vi "GetDataEvent_Service_3.vi"() -> ()   [LabVIEW 2017]
doc: "This is an example of how to read Data Sets from the InsightCM database. Using a similiar method you can read any waveform that has been stored and perform additional analysis on it or save it to a file format."
uses:
  <vilib>/addons/InsightCM/MessageBus/Base/controls/AssetNodeView.ctl
  <vilib>/addons/InsightCM/MessageBus/Base/controls/AssetState.ctl
  <vilib>/addons/InsightCM/MessageBus/Base/controls/Metric.ctl
  <vilib>/addons/InsightCM/MessageBus/Base/controls/KeyValuePair.ctl
  <vilib>/addons/InsightCM/MessageBus/Base/controls/AssetNodeReference.ctl
  <vilib>/addons/InsightCM/MessageBus/Base/controls/DataEvent.ctl
  <vilib>/addons/InsightCM/MessageBus/Base/controls/DataSetByteData.ctl
  <vilib>/addons/InsightCM/MessageBus/Base/controls/TrendPoint.ctl
  typedefs/Asset Info.ctl
  typedefs/Sensor Info.ctl
  typedefs/Metric Info.ctl
  typedefs/Q_Message.ctl
  typedefs/Input IDs.ctl
  <vilib>/addons/InsightCM/MessageBus/MessageService/IcmMessageService.lvclass
panel:
  out "element":T1
  out "Output 2":T2(array[cluster])
  out "DataEvents 2":T3[](array[typedef])=[{"Id"="{6C8D9120-E97A-11E9-9C35-00802F195E7B}", "AssetNodeId"="5cf73cf3a0991c03a125caeb", "Timestamp"=1570418361, "Props"=[{"Key"="DeviceName", "Value"="John-9068"}, {"Key"="DataGroup", "Value"="Equipment"}, {"Key"="OpState", "Value"="Default"}, {"Key"="Reason", "Value"="User Event"}, {"Key"="HighRate", "Value"="true"}, {"Key"="HasDataSets", "Value"="true"}]}, {"Id"="{7F637499-E981-11E9-A30F-00802F195E7B}", "AssetNodeId"="5cf73cf3a0991c03a125caeb", "Timestamp"=1570421399, "Props"=[{"Key"="DeviceName", "Value"="John-9068"}, {"Key"="DataGroup", "Value"="Equipment"}, {"Key"="OpState", "Value"="Default"}, {"Key"="Reason", "Value"="Periodic Event"}, {"Key"="HighRate", "Value"="true"}, {"Key"="HasDataSets", "Value"="true"}]}, {"Id"="{E4F320D8-E982-11E9-A025-00802F195E7B}", "AssetNodeId"="5cf73cf3a0991c03a125caeb", "Timestamp"=1570421999, "Props"=[{"Key"="DeviceName", "Value"="John-9068"}, {"Key"="DataGroup", "Value"="Equipment"}, {"Key"="OpState", "Value"="Default"}, {"Key"="Reason", "Value"="Periodic Event"}, {"Key"="HighRate", "Value"="true"}, {"Key"="HasDataSets", "Value"="true"}]}, {"Id"="{97B5DB2B-E983-11E9-8698-00802F195E7B}", "AssetNodeId"="5cf73cf3a0991c03a125caeb", "Timestamp"=1570422299, "Props"=[{"Key"="DeviceName", "Value"="John-9068"}, {"Key"="DataGroup", "Value"="Equipment"}, {"Key"="OpState", "Value"="Default"}, {"Key"="Reason", "Value"="Periodic Event"}, {"Key"="HighRate", "Value"="true"}, {"Key"="HasDataSets", "Value"="true"}]}, {"Id"="{FD7A4AB0-E984-11E9-A552-00802F195E7B}", "AssetNodeId"="5cf73cf3a0991c03a125caeb", "Timestamp"=1570422899, "Props"=[{"Key"="DeviceName", "Value"="John-9068"}, {"Key"="DataGroup", "Value"="Equipment"}, {"Key"="OpState", "Value"="Default"}, {"Key"="Reason", "Value"="Periodic Event"}, {"Key"="HighRate", "Value"="true"}, {"Key"="HasDataSets", "Value"="true"}]}, {"Id"="{B025F119-E985-11E9-9683-00802F195E7B}", "AssetNodeId"="5cf73cf3a0991c03a125caeb", "Timestamp"=1570423199, "Props"=[{"Key"="DeviceName", "Value"="John-9068"}, {"Key"="DataGroup", "Value"="Equipment"}, {"Key"="OpState", "Value"="Default"}, {"Key"="Reason", "Value"="Periodic Event"}, {"Key"="HighRate", "Value"="true"}, {"Key"="HasDataSets", "Value"="true"}]}, {"Id"="{62F87800-E986-11E9-9683-00802F195E7B}", "AssetNodeId"="5cf73cf3a0991c03a125caeb", "Timestamp"=1570423499, "Props"=[{"Key"="DeviceName", "Value"="John-9068"}, {"Key"="DataGroup", "Value"="Equipment"}, {"Key"="OpState", "Value"="Default"}, {"Key"="Reason", "Value"="Periodic Event"}, {"Key"="HighRate", "Value"="true"}, {"Key"="HasDataSets", "Value"="true"}]}]
  out "LastTrendPoint":cluster{string, "Value":dbl}
  in  "String":string="This is an EXE to host a web service for InsightCM.\n\nhttp://127.0.0.1:8002/Query/GetLastEvent?Asset=<AssetName>\nOutput: Last event for the asset within X days, all channels (JSON)\n\nhttp://127.0.0.1:8002/Query/GetAssetList\nOutput: Asset ID, Sensor ID, and Metric ID (JSON)\n\nhttp://127.0.0.1:8002/Query/GetLastTrend?MetricID=<Metric ID of feature>\nOutput: Time and value of last trend point (JSON)\n\nhttp://127.0.0.1:8002/Query/GetEventList?FID_2={value}&FID_1={value}&SensorID={value}&AssetID={value}\nOutput: From asset and sensor, give list of recent event waveform and feature data (JSON)\n\nhttp://127.0.0.1:8002/Query/GetEvent?FID_2={value}&FID_1={value}&SensorID={value}&AssetID={value}\nOutput: From asset and sensor, give most recent event waveform and feature data (JSON)"
  out "Trend":T5(graph)
  out "SIGMU Output":T6[](array[typedef])
  in  "Seconds from now":i64=3600
  out "error out":errorcluster
  out "Ready?":bool
  out "Parameter (debug)":string
  out "Command (debug)":string
  out "Output":T9(array[cluster])
  out "TrendPoints":T10[](array[typedef])
  out "DataSets":T11[](array[typedef])
  out "date/time":string
  out "Numeric":i32
  out "DataEvents":T3[](array[typedef])
  out "AssetNodeView":T12
  out "AssetNodes":T12[](array[typedef])
  # "1 hr = 3600, 1 day = 86400"
  # "This example shows how to query InsightCM data.\n\n1) Click Refresh to load assets.\n2) Select an asset.\n3) Select a data event and a sensor.\n\nNote: If the sensor does not have waveform data, the waveform graph will be empty."
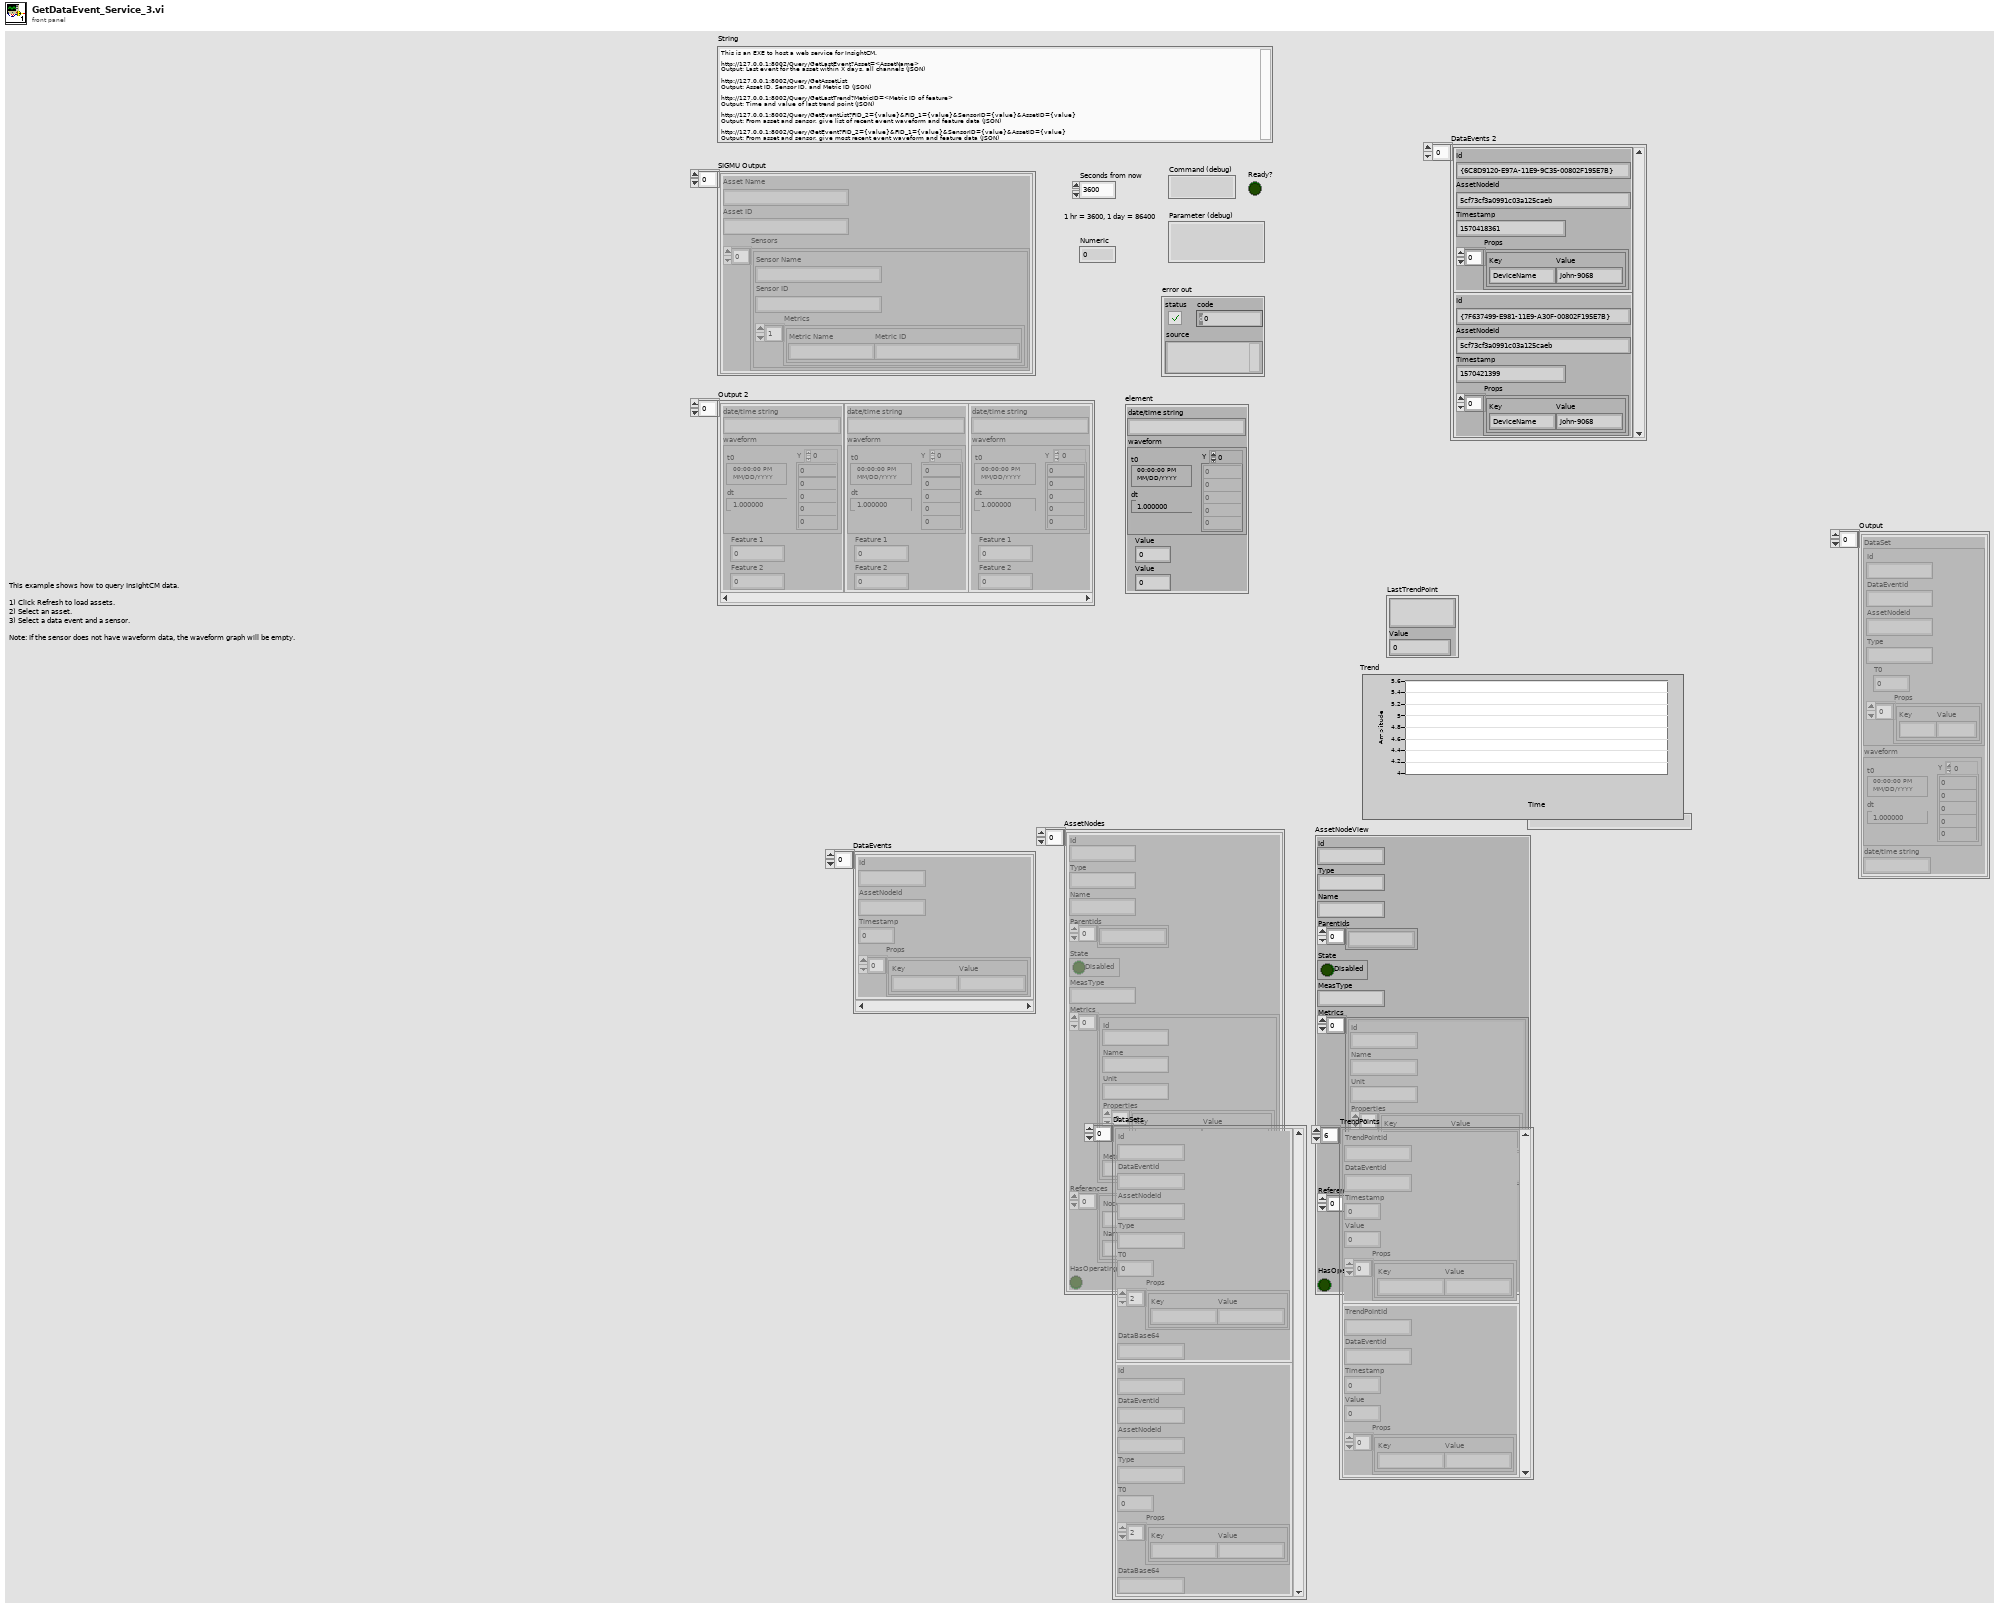
[diagram p1: front panel]
types:
  T1 = cluster{"date/time string":string, "waveform":waveform(sgl), "Value":dbl, "Value":dbl}
  T2 = cluster{"date/time string":string, "waveform":waveform(sgl), "Feature 1":dbl, "Feature 2":dbl}[]
  T3 = typedef "DataEvent.ctl" = cluster{"Id":string, "AssetNodeId":string, "Timestamp":i64, "Props":T4[]}
  T4 = typedef "KeyValuePair.ctl" = cluster{"Key":string, "Value":string}
  T5 = cluster{"Time Stamp out":timestamp, "Value":dbl}[]
  T6 = typedef "Asset Info.ctl" = cluster{"Asset Name":string, "Asset ID":string, "Sensors":T7[]}
  T7 = typedef "Sensor Info.ctl" = cluster{"Sensor Name":string, "Sensor ID":string, "Metrics":T8[]}
  T8 = typedef "Metric Info.ctl" = cluster{"Metric Name ":string, "Metric ID":string}
  T9 = cluster{"DataSet":cluster{"Id":string, "DataEventId":string, "AssetNodeId":string, "Type":string, "T0":i64, "Props":T4[]}, "waveform":waveform(sgl), "date/time string":string}[]
  T10 = typedef "TrendPoint.ctl" = cluster{"TrendPointId":string, "DataEventId":string, "Timestamp":i64, "Value":dbl, "Props":T4[]}
  T11 = typedef "DataSetByteData.ctl" = cluster{"Id":string, "DataEventId":string, "AssetNodeId":string, "Type":string, "T0":i64, "Props":T4[], "DataBase64":string}
  T12 = typedef "AssetNodeView.ctl" = cluster{"Id":string, "Type":string, "Name":string, "ParentIds":string[], "State":T13, "MeasType":string, "Metrics":T14[], "References":T15[], "HasOperatingStates":bool}
  T13 = typedef "AssetState.ctl" = cluster{"Disabled":bool}
  T14 = typedef "Metric.ctl" = cluster{"Id":string, "Name":string, "Unit":string, "Properties":T4[], "MetricDefinitionInstanceId":string}
  T15 = typedef "AssetNodeReference.ctl" = cluster{"NodeId":string, "Name":string}
  T16 = typedef "Q_Message.ctl" = cluster{"Command":string, "Parameters":variant}
  T17 = cluster{"Id":string, "DataEventId":string, "AssetNodeId":string, "Type":string, "T0":i64, "Props":T4[]}
  T18 = cluster{"DataSet":cluster{"Id":string, "DataEventId":string, "AssetNodeId":string, "Type":string, "T0":i64, "Props":T4[]}, "waveform":waveform(sgl), "date/time string":string}
  T19 = typedef "Input IDs.ctl" = cluster{"Asset ID":string, "Sensor ID":string, "Feature id 1":string, "Feature id 2":string}
  T20 = cluster{"date/time string":string, "waveform":waveform(sgl), "Value":dbl, "Value":dbl}[]
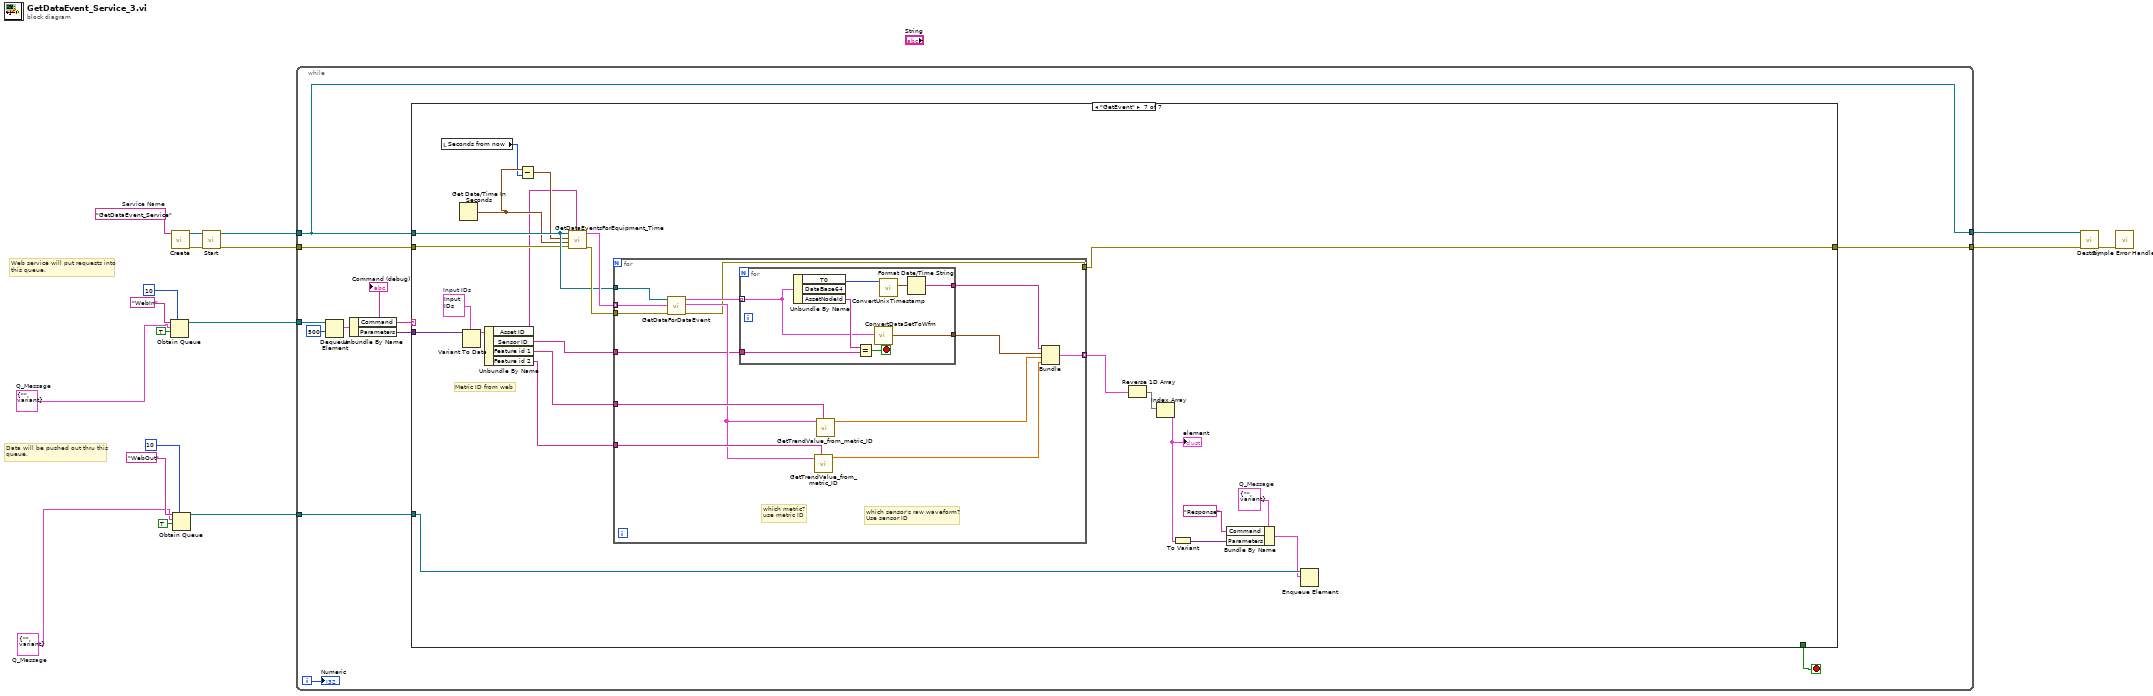
[diagram p0: block diagram]
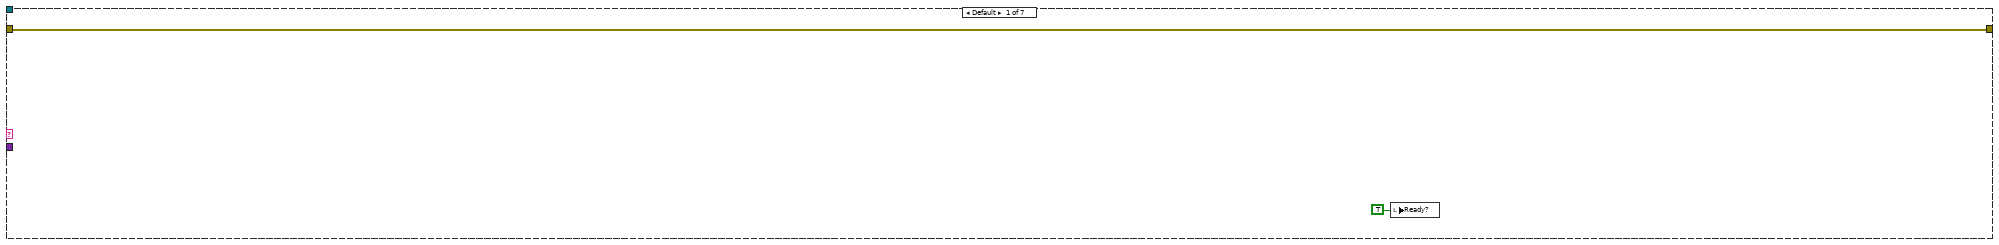
[diagram p2: hidden frame]
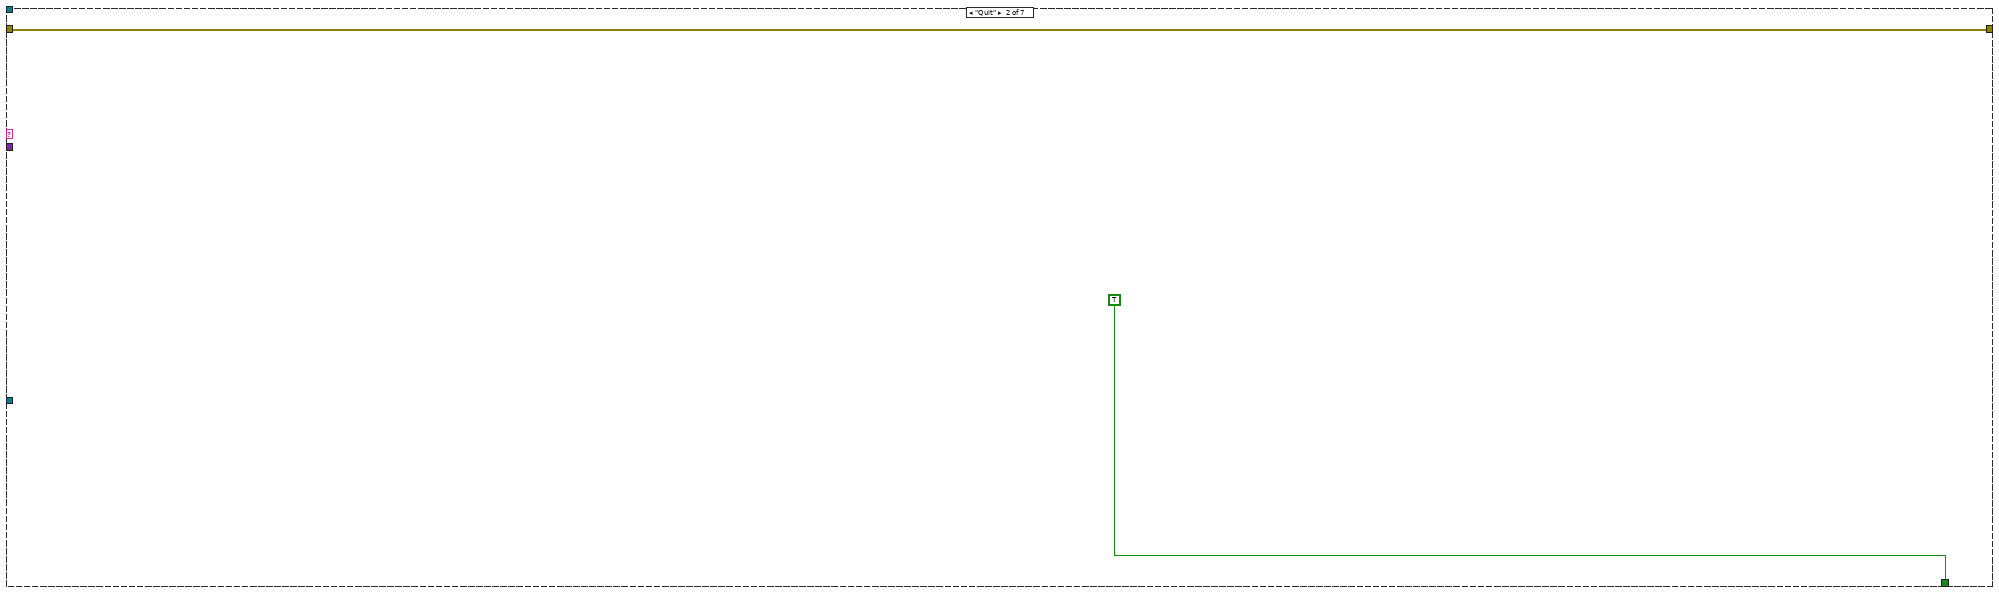
[diagram p3: hidden frame]
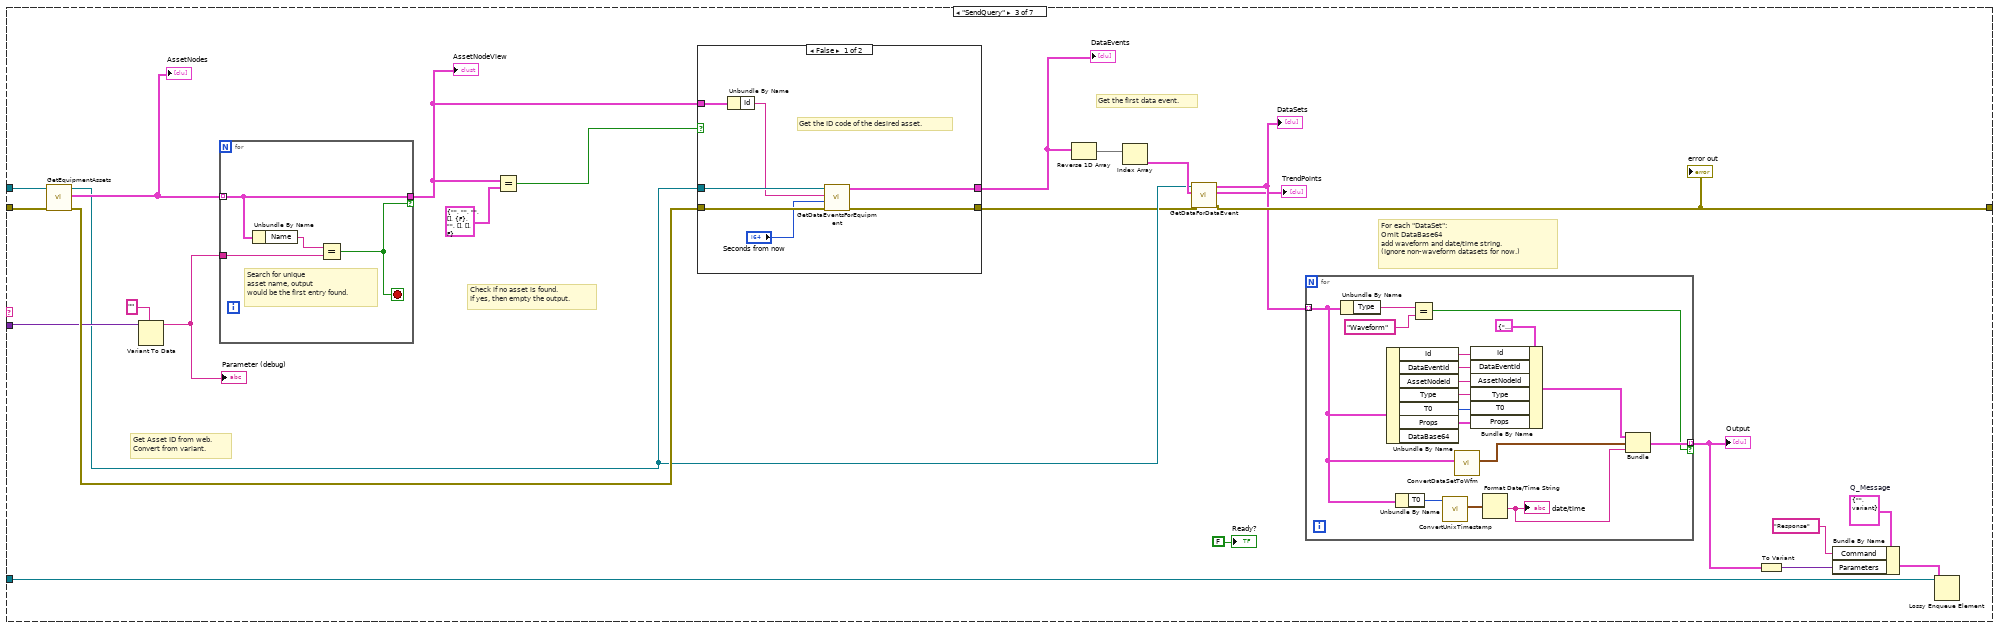
[diagram p4: hidden frame]
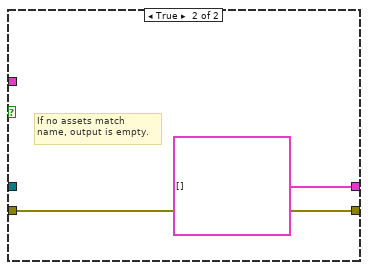
[diagram p5: hidden frame]
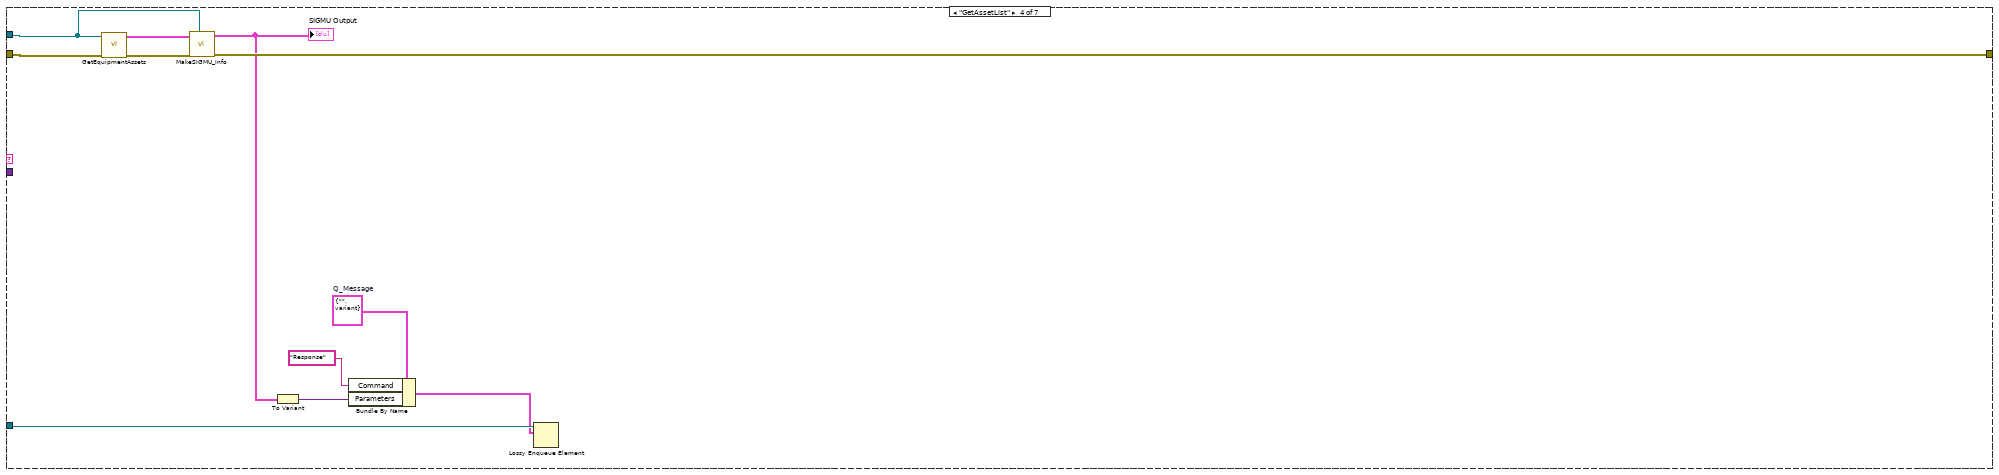
[diagram p6: hidden frame]
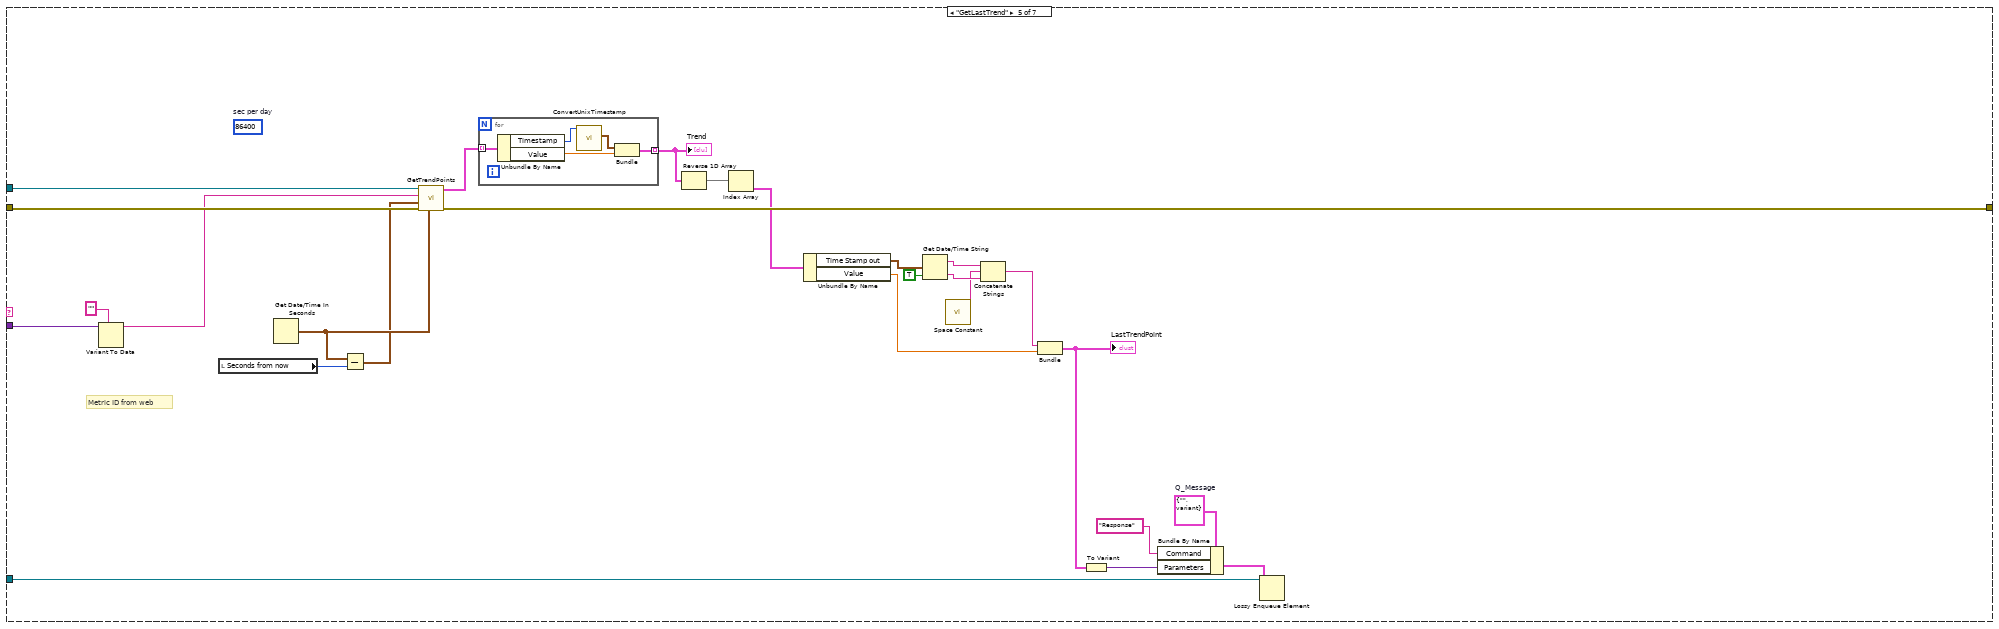
[diagram p7: hidden frame]
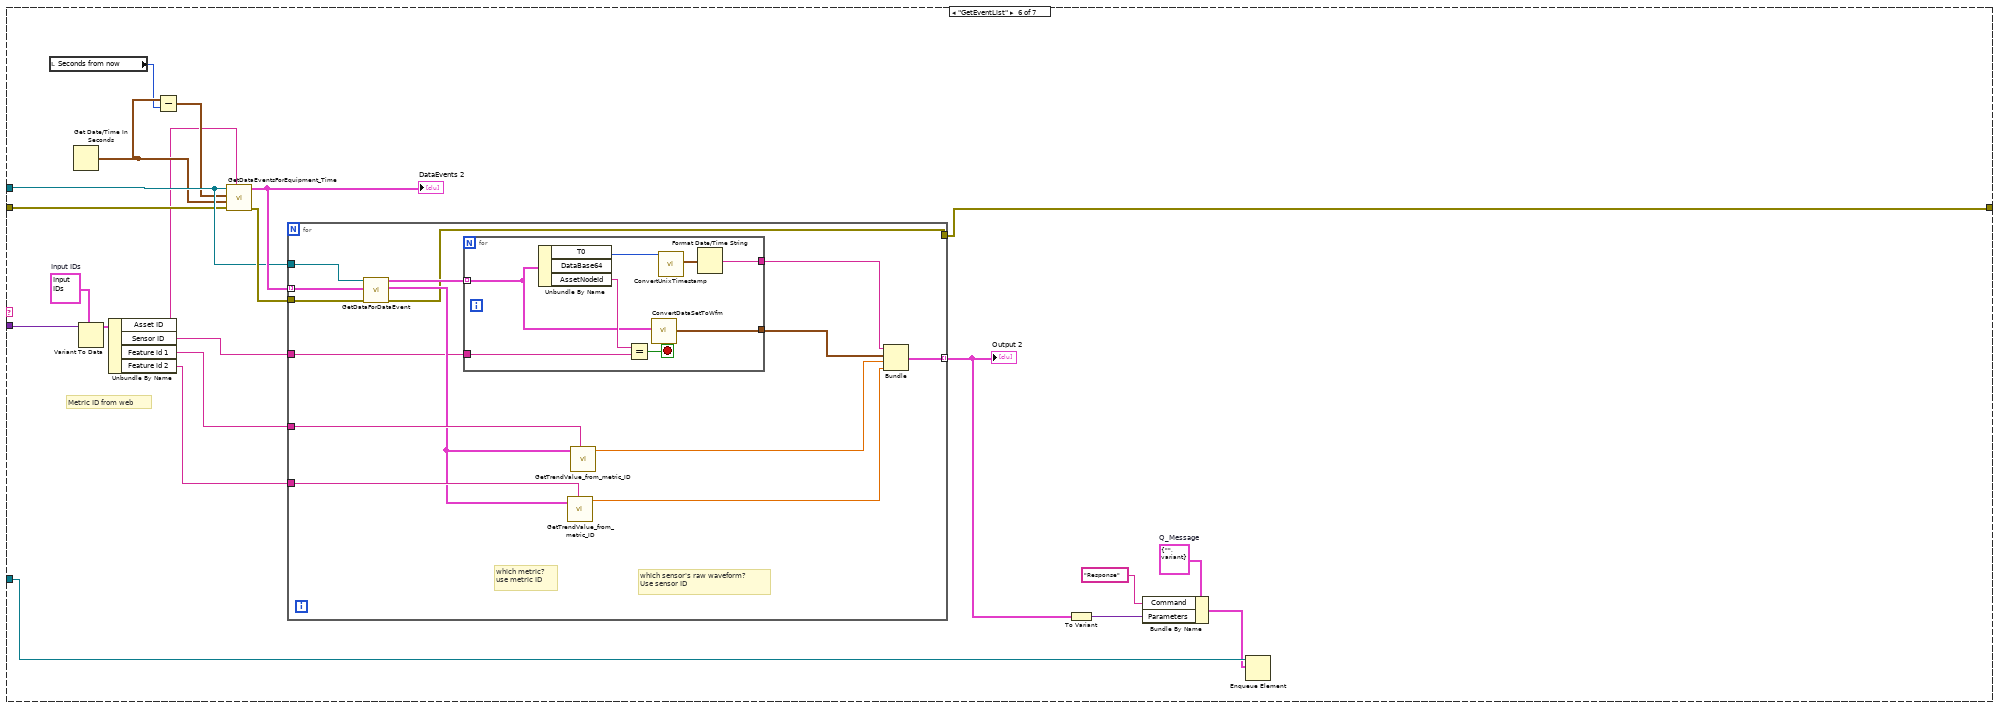
[diagram p8: hidden frame]
diagram:
  w1 = T16 {"Command"="", "Parameters"=variant}  # Q_Message
  w2 = T16 {"Command"="", "Parameters"=variant}  # Q_Message
  w18 = "GetDataEvent_Service"  # Service Name
  # "Data will be pushed out thru this\nqueue."
  # "Web service will put requests into\nthis queue."
  n1 = Obtain Queue(max queue size (-1, unlimited)=10, name (unnamed)="WebIn", element data type=w2, create if not found? (T)=TRUE) -> (queue out=w8:refnum<queue>)  [unwired: 1 in, 2 out]
  n2 = call <vilib>:"Create.vi"("service name"=w18) -> ("error out"=w13:errorcluster, "service out"=w14:refnum<class "IcmMessageService.lvclass">)  [unwired: 9 in]
  n3 = Obtain Queue(max queue size (-1, unlimited)=10, name (unnamed)="WebOut", element data type=w1, create if not found? (T)=TRUE) -> (queue out=w7:refnum<queue>)  [unwired: 1 in, 2 out]
  n4 = call <vilib>:"Start.vi"("error in (no error)"=w13, "service in"=w14) -> ("error out"=w11:errorcluster, "service out"=w12:refnum<class "IcmMessageService.lvclass">)  [unwired: 8 in]
  n5 = while {
    tunnel: w12 -> [w28]
    tunnel: w11 -> [w29]
    tunnel: [w28] -> w15
    tunnel: [w27] -> w16
    tunnel: w8 -> [w26]
    tunnel: w7 -> [w24]
    i -> [w19]
    stop <- w23 stop-if-true
    n6 = Dequeue Element(queue=w26, timeout in ms (-1)=500) -> (element=w22:T16)  [unwired: 1 in, 3 out]
    n7 = Unbundle By Name(w22) -> ("Command"=w21:string, "Parameters"=w20:variant)
    "Command (debug)" <- w21
    n8 = case shown="\"GetEvent\"" w21 {
      tunnel: w29 -> [w31 w33 w57 w98 w122 w147 w192]
      tunnel: w28 -> [_ _ w45 w96 w123 w148 w193]
      tunnel: [w31 w33 w43 w94 w115 w130 w176] -> w27
      tunnel: w24 -> [_ _ w36 w90 w108 w136 w181]
      tunnel: [_ TRUE _ _ _ _ _] -> w23
      tunnel: w20 -> [_ _ w51 _ w120 w146 w191]
      frame Default {
        n9 = local write "Ready?"(TRUE ("Ready?")) -> ()
      }
      frame "Quit" {
      }
      frame "SendQuery" {
        w34 = T16 {"Command"="", "Parameters"=variant}  # Q_Message
        # "For each \"DataSet\":\nOmit DataBase64\nadd waveform and date/time string.\n(Ignore non-waveform datasets for now.)"
        # "Get Asset ID from web.\nConvert from variant."
        # "Get the first data event."
        # "Check if no asset is found.\nIf yes, then empty the output."
        n10 = call "GetEquipmentAssets.vi"("error in (no error)"=w57, "service"=w45) -> ("error out"=w53:errorcluster, "AssetNodes"=w56:T12[])  [unwired: 8 in]
        "AssetNodes" <- w56
        n11 = Variant To Data(type="", Variant=w51) -> (data=w49:string)  [unwired: 1 in, 1 out]
        "Parameter (debug)" <- w49
        n12 = for {
          tunnel: w56 -> [w85] mode=indexing
          tunnel: w49 -> [w86]
          tunnel: [w85] -> w54 if=w84
          stop <- w84 stop-if-true
          # "Search for unique \nasset name, output\nwould be the first entry found."
          n13 = Unbundle By Name(w85) -> ("Name"=w87:string)
          n14 = Equal?(x=w87, y=w86) -> (x = y?=w84:bool)
        }
        "AssetNodeView" <- w54
        n15 = Equal?(x=w54, y=T12 {"Id"="", "Type"="", "Name"="", "ParentIds"=[], "State"={"Disabled"=FALSE}, "MeasType"="", "Metrics"=[], "References"=[], "HasOperatingStates"=FALSE} ("AssetNodeView 2")) -> (x = y?=w52:bool)
        n16 = case shown="False" w52 {
          tunnel: w54 -> [w79 _]
          tunnel: w45 -> [w81 _]
          tunnel: w53 -> [w80 w82]
          tunnel: [w78 T3[] [] ("DataEvents")] -> w48
          tunnel: [w77 w82] -> w44
          frame False {
            # "Get the ID code of the desired asset."
            n17 = Unbundle By Name(w79) -> ("Id"=w76:string)
            n18 = call "GetDataEventsForEquipment.vi"("error in (no error)"=w80, "sec per day"="Seconds from now", "equipment id"=w76, "service"=w81) -> ("error out"=w77:errorcluster, "DataEvents"=w78:T3[])  [unwired: 6 in]
          }
          frame True {
            # "If no assets match\nname, output is empty."
          }
        }
        "DataEvents" <- w48
        n19 = Reverse 1D Array(array=w48) -> (reversed array=w47:T3[])
        n20 = Index Array(array=w47) -> (element=w46:T3)  [unwired: 1 in]
        n21 = call "GetDataForDataEvent.vi"("error in (no error)"=w44, "DataEvent"=w46, "service"=w45) -> ("error out"=w43:errorcluster, "TrendPoints"=→"TrendPoints":T10[], "DataSets"=w42:T11[])  [unwired: 6 in]
        "DataSets" <- w42
        "error out" <- w43
        n22 = for {
          tunnel: w42 -> [w66] mode=indexing
          tunnel: [w68] -> w35 mode=indexing if=w67
          n23 = Unbundle By Name(w66) -> ("Type"=w74:string)
          n24 = Unbundle By Name(w66) -> ("Id"=w64:string, "DataEventId"=w60:string, "AssetNodeId"=w61:string, "Type"=w62:string, "T0"=w63:i64, "Props"=w59:T4[])  [unwired: 1 out]
          n25 = Unbundle By Name(w66) -> ("T0"=w72:i64)
          n26 = Equal?(x=w74, y="Waveform") -> (x = y?=w67:bool)
          n27 = call <vilib>:"ConvertUnixTimestamp.vi"("Timestamp in"=w72) -> ("Time Stamp out"=w71:timestamp)  [unwired: 10 in]
          n28 = call "ConvertDataSetToWfm.vi"("DataSet"=w66) -> ("waveform"=w70:waveform(sgl))  [unwired: 10 in]
          n29 = Bundle By Name(cluster=T17 {"Id"="", "DataEventId"="", "AssetNodeId"="", "Type"="", "T0"=0, "Props"=[]} ("DataSet"), "Id"=w64, "DataEventId"=w60, "AssetNodeId"=w61, "Type"=w62, "T0"=w63, "Props"=w59) -> (w58:T17)
          n30 = Format Date/Time String(seconds (now)=w71) -> (date/time string=w69:string)  [unwired: 2 in]
          "date/time" <- w69
          n31 = Bundle("DataSet"=w58, "waveform"=w70, "date/time string"=w69) -> (w68:T18)  [unwired: 1 in]
        }
        "Output" <- w35
        n32 = To Variant(anything=w35) -> (Variant=w38:variant)
        n33 = Bundle By Name(cluster=w34, "Command"="Response", "Parameters"=w38) -> (w37:T16)
        n34 = Lossy Enqueue Element(queue=w36, element=w37) -> ()  [unwired: 1 in, 4 out]
        "Ready?" <- FALSE ("Ready?")
      }
      frame "GetAssetList" {
        w88 = T16 {"Command"="", "Parameters"=variant}  # Q_Message
        n35 = call "GetEquipmentAssets.vi"("error in (no error)"=w98, "service"=w96) -> ("error out"=w95:errorcluster, "AssetNodes"=w97:T12[])  [unwired: 8 in]
        n36 = call "MakeSIGMU_Info.vi"("ICM Service in"=w96, "error in (no error)"=w95, "AssetNodes In"=w97) -> ("error out"=w94:errorcluster, "SIGMU Output"=w93:T6[])  [unwired: 7 in]
        "SIGMU Output" <- w93
        n37 = To Variant(anything=w93) -> (Variant=w91:variant)
        n38 = Bundle By Name(cluster=w88, "Command"="Response", "Parameters"=w91) -> (w89:T16)
        n39 = Lossy Enqueue Element(queue=w90, element=w89) -> ()  [unwired: 1 in, 4 out]
      }
      frame "GetLastTrend" {
        w109 = T16 {"Command"="", "Parameters"=variant}  # Q_Message
        (unwired) 86400  # sec per day
        # "Metric ID from web"
        n40 = Variant To Data(type="", Variant=w120) -> (data=w119:string)  [unwired: 1 in, 1 out]
        n41 = local read "Seconds from now"() -> (w117:i64)
        n42 = Get Date/Time In Seconds() -> (seconds since 1Jan1904=w118:timestamp)
        n43 = Subtract(x=w118, y=w117) -> (x-y=w116:timestamp)
        n44 = call "GetTrendPoints.vi"("End Time"=w118, "error in (no error)"=w122, "Start Time"=w116, "trend id"=w119, "service"=w123) -> ("error out"=w115:errorcluster, "TrendPoints"=w124:T10[])  [unwired: 5 in]
        n45 = for {
          tunnel: w124 -> [w129] mode=indexing
          tunnel: [w128] -> w113 mode=indexing
          n46 = Unbundle By Name(w129) -> ("Timestamp"=w126:i64, "Value"=w127:dbl)
          n47 = call <vilib>:"ConvertUnixTimestamp.vi"("Timestamp in"=w126) -> ("Time Stamp out"=w125:timestamp)  [unwired: 10 in]
          n48 = Bundle("Time Stamp out"=w125, "Value"=w127) -> (w128:cluster{"Time Stamp out":timestamp, "Value":dbl})  [unwired: 1 in]
        }
        "Trend" <- w113
        n49 = Reverse 1D Array(array=w113) -> (reversed array=w114:T5)
        n50 = Index Array(array=w114) -> (element=w100:cluster{"Time Stamp out":timestamp, "Value":dbl})  [unwired: 1 in]
        n51 = Unbundle By Name(w100) -> ("Time Stamp out"=w107:timestamp, "Value"=w101:dbl)
        n52 = Get Date/Time String(seconds (now)=w107, want seconds? (F)=TRUE) -> (date string=w105:string, time string=w104:string)  [unwired: 1 in]
        n53 = call <vilib>:"Space Constant.vi"() -> ("String"=w103:string)
        n54 = Concatenate Strings(w105, w103, w104) -> (w102:string)
        n55 = Bundle(w102, "Value"=w101) -> (w99:cluster{string, "Value":dbl})  [unwired: 1 in]
        "LastTrendPoint" <- w99
        n56 = To Variant(anything=w99) -> (Variant=w111:variant)
        n57 = Bundle By Name(cluster=w109, "Command"="Response", "Parameters"=w111) -> (w110:T16)
        n58 = Lossy Enqueue Element(queue=w108, element=w110) -> ()  [unwired: 1 in, 4 out]
      }
      frame "GetEventList" {
        w133 = T16 {"Command"="", "Parameters"=variant}  # Q_Message
        w142 = T19 {"Asset ID"="5cf73cf3a0991c03a125caeb", "Sensor ID"="5cf73d1ba0991c03a125caee", "Feature id 1"="5cf73d1ba0991c03a125caef", "Feature id 2"="5cf73d1ba0991c03a125caf0"}  # Input IDs
        # "Metric ID from web"
        n59 = local read "Seconds from now"() -> (w144:i64)
        n60 = Get Date/Time In Seconds() -> (seconds since 1Jan1904=w145:timestamp)
        n61 = Variant To Data(type=w142, Variant=w146) -> (data=w141:T19)  [unwired: 1 in, 1 out]
        n62 = Unbundle By Name(w141) -> ("Asset ID"=w140:string, "Sensor ID"=w137:string, "Feature id 1"=w138:string, "Feature id 2"=w139:string)
        n63 = Subtract(x=w145, y=w144) -> (x-y=w143:timestamp)
        n64 = call "GetDataEventsForEquipment_Time.vi"("equipment id"=w140, "error in (no error)"=w147, "End Time"=w145, "Start Time"=w143, "service"=w148) -> ("error out"=w150:errorcluster, "DataEvents"=w149:T3[])  [unwired: 5 in]
        "DataEvents 2" <- w149
        n65 = for {
          tunnel: w148 -> [w164]
          tunnel: w150 -> [w163]
          tunnel: w149 -> [w162] mode=indexing
          tunnel: [w157] -> w132 mode=indexing
          tunnel: w138 -> [w156]
          tunnel: w139 -> [w155]
          tunnel: w137 -> [w152]
          tunnel: [w151] -> w130
          # "which metric?\nuse metric ID"
          # "which sensor's raw waveform?\nUse sensor ID"
          n66 = call "GetDataForDataEvent.vi"("error in (no error)"=w163, "DataEvent"=w162, "service"=w164) -> ("error out"=w151:errorcluster, "TrendPoints"=w154:T10[], "DataSets"=w161:T11[])  [unwired: 6 in]
          n67 = for {
            tunnel: w161 -> [w167] mode=indexing
            tunnel: w152 -> [w171]
            tunnel: [w166] -> w160
            tunnel: [w165] -> w159
            stop <- w170 stop-if-true
            n68 = Unbundle By Name(w167) -> ("T0"=w168:i64, "AssetNodeId"=w172:string)  [unwired: 1 out]
            n69 = Equal?(x=w172, y=w171) -> (x = y?=w170:bool)
            n70 = call "ConvertDataSetToWfm.vi"("DataSet"=w167) -> ("waveform"=w165:waveform(sgl))  [unwired: 10 in]
            n71 = call <vilib>:"ConvertUnixTimestamp.vi"("Timestamp in"=w168) -> ("Time Stamp out"=w169:timestamp)  [unwired: 10 in]
            n72 = Format Date/Time String(seconds (now)=w169) -> (date/time string=w166:string)  [unwired: 2 in]
          }
          n73 = call "GetTrendValue_from_metric_ID.vi"("Input: trend id"=w155, "TrendPoints"=w154) -> ("Value"=w153:dbl)  [unwired: 9 in]
          n74 = call "GetTrendValue_from_metric_ID.vi"("Input: trend id"=w156, "TrendPoints"=w154) -> ("Value"=w158:dbl)  [unwired: 9 in]
          n75 = Bundle("date/time string"=w160, "waveform"=w159, "Value"=w158, "Value"=w153) -> (w157:T1)  [unwired: 1 in]
        }
        "Output 2" <- w132
        n76 = To Variant(anything=w132) -> (Variant=w134:variant)
        n77 = Bundle By Name(cluster=w133, "Command"="Response", "Parameters"=w134) -> (w131:T16)
        n78 = Enqueue Element(queue=w136, element=w131) -> ()  [unwired: 2 in, 3 out]
      }
      frame "GetEvent" {
        w178 = T16 {"Command"="", "Parameters"=variant}  # Q_Message
        w187 = T19 {"Asset ID"="5cf73cf3a0991c03a125caeb", "Sensor ID"="5cf73d1ba0991c03a125caee", "Feature id 1"="5cf73d1ba0991c03a125caef", "Feature id 2"="5cf73d1ba0991c03a125caf0"}  # Input IDs
        # "Metric ID from web"
        n79 = local read "Seconds from now"() -> (w189:i64)
        n80 = Get Date/Time In Seconds() -> (seconds since 1Jan1904=w190:timestamp)
        n81 = Variant To Data(type=w187, Variant=w191) -> (data=w186:T19)  [unwired: 1 in, 1 out]
        n82 = Unbundle By Name(w186) -> ("Asset ID"=w185:string, "Sensor ID"=w182:string, "Feature id 1"=w183:string, "Feature id 2"=w184:string)
        n83 = Subtract(x=w190, y=w189) -> (x-y=w188:timestamp)
        n84 = call "GetDataEventsForEquipment_Time.vi"("equipment id"=w185, "error in (no error)"=w192, "End Time"=w190, "Start Time"=w188, "service"=w193) -> ("error out"=w195:errorcluster, "DataEvents"=w194:T3[])  [unwired: 5 in]
        n85 = for {
          tunnel: w193 -> [w209]
          tunnel: w195 -> [w208]
          tunnel: w194 -> [w207] mode=indexing
          tunnel: [w202] -> w175 mode=indexing
          tunnel: w183 -> [w201]
          tunnel: w184 -> [w200]
          tunnel: w182 -> [w197]
          tunnel: [w196] -> w176
          # "which metric?\nuse metric ID"
          # "which sensor's raw waveform?\nUse sensor ID"
          n86 = call "GetDataForDataEvent.vi"("error in (no error)"=w208, "DataEvent"=w207, "service"=w209) -> ("error out"=w196:errorcluster, "TrendPoints"=w199:T10[], "DataSets"=w206:T11[])  [unwired: 6 in]
          n87 = for {
            tunnel: w206 -> [w212] mode=indexing
            tunnel: w197 -> [w216]
            tunnel: [w211] -> w205
            tunnel: [w210] -> w204
            stop <- w215 stop-if-true
            n88 = Unbundle By Name(w212) -> ("T0"=w213:i64, "AssetNodeId"=w217:string)  [unwired: 1 out]
            n89 = Equal?(x=w217, y=w216) -> (x = y?=w215:bool)
            n90 = call "ConvertDataSetToWfm.vi"("DataSet"=w212) -> ("waveform"=w210:waveform(sgl))  [unwired: 10 in]
            n91 = call <vilib>:"ConvertUnixTimestamp.vi"("Timestamp in"=w213) -> ("Time Stamp out"=w214:timestamp)  [unwired: 10 in]
            n92 = Format Date/Time String(seconds (now)=w214) -> (date/time string=w211:string)  [unwired: 2 in]
          }
          n93 = call "GetTrendValue_from_metric_ID.vi"("Input: trend id"=w200, "TrendPoints"=w199) -> ("Value"=w198:dbl)  [unwired: 9 in]
          n94 = call "GetTrendValue_from_metric_ID.vi"("Input: trend id"=w201, "TrendPoints"=w199) -> ("Value"=w203:dbl)  [unwired: 9 in]
          n95 = Bundle("date/time string"=w205, "waveform"=w204, "Value"=w203, "Value"=w198) -> (w202:T1)  [unwired: 1 in]
        }
        n96 = Reverse 1D Array(array=w175) -> (reversed array=w174:T20)
        n97 = Index Array(array=w174) -> (element=w173:T1)  [unwired: 1 in]
        "element" <- w173
        n98 = To Variant(anything=w173) -> (Variant=w179:variant)
        n99 = Bundle By Name(cluster=w178, "Command"="Response", "Parameters"=w179) -> (w177:T16)
        n100 = Enqueue Element(queue=w181, element=w177) -> ()  [unwired: 2 in, 3 out]
      }
    }
    "Numeric" <- w19
  }
  n101 = call <vilib>:"Destroy.vi"("error in (no error)"=w16, "service in"=w15) -> ("error out"=w17:errorcluster)  [unwired: 9 in]
  n102 = call <vilib>:"Simple Error Handler.vi"("error in (no error)"=w17) -> ()  [unwired: 4 in, 5 out]
